vi "Positioncontrol_twomotor_pid_PMcheck.vi"() -> ()   [LabVIEW 2014]
uses:
  <vilib>/rvi/FXPMathLib/FxpSinAndCos/subVIs/nifxpmath_SinAndCos_SimConfig.ctl
  <vilib>/rvi/Emulation/niFpgaGetClockAttributes.vi
  <vilib>/rvi/Emulation/niFpgaSctlEmulationGetInTimedLoop.vi
  <vilib>/rvi/Emulation/niFpgaEmulationReportErrorSimple.vi
  <vilib>/rvi/Emulation/niFpgaProcessEmulError.vi
  <vilib>/rvi/FXPMathLib/FxpSinAndCos/simVIs/DllFxpSinAndCosTemp_sub.vi
  <vilib>/rvi/Emulation/niFpgaCriticalErrorInLSC.vi
  <vilib>/rvi/eio/common/nirviEmuTemplateMethod_errors.vi
  <vilib>/rvi/interface/RandomDataEmulation/nirviRandomDataMultiElementFPGAFIFO.vi
  <instcachedir>/0/nirviRandomDataMultiElementFPGAFIFO_AD0CFC12EF974623A9C2E4184BC062B2.lvgen/nirviRandomDataMultiElementFPGAFIFO_AD0CFC12EF974623A9C2E4184BC062B2_004.vi
  <vilib>/rvi/interface/RandomDataEmulation/niFpgaRandomDataHandleErrors.vi
  <vilib>/rvi/FXPMathLib/FxpSinAndCos/XNode/nifxpmath_SinAndCos.xnode
  <vilib>/eio/EIONode/EIONode.xnode
  <vilib>/rvi/FXPMathLib/FxpMul/XNode/nifxpmath_Multiplier.xnode
  <vilib>/rvi/FXPMathLib/FxpSub/XNode/nifxpmath_Sub.xnode
  <vilib>/rvi/FXPMathLib/FxpAdd/XNode/nifxpmath_Add.xnode
  <vilib>/rvi/Analysis/measure/butterworth/XNode/niFpgaButterworthFilter.xnode
  <vilib>/rvi/DataTransferAndStorage/Container/XNode/niFpgaContainer.xnode
  <vilib>/rvi/interface/RandomDataEmulation/nirviRandomDataFpgaMultiElementTemplate.vi
  <vilib>/rvi/FXPMathLib/sim/FxpSim.dll
panel:
  in  "AI loop wait (uSec)":u8=20
  in  "x_y 2 / x_y":bool
  in  "test stop/run":bool
  out "AI samp time (us) 3":u8
  in  "scaled coefficients_xy":i32[](array[numeric])=[-955995012, 2025731616, 1001305, -1023351008, 2092954700, 1034533]
  in  "scaled coefficients_xyd":i32[](array[numeric])=[-1013179863, 2085891919, 257442, -1048234864, 2120929620, 261767]
  in  "filter reset 2":bool
  out "AI diff samp time (us) 2":u8
  in  "AI diff loop wait (uSec) 2":u32
  out "Dy_d 2":fxp<+/-,25,15>
  out "Dp_d 2":fxp<+/-,25,15>
  in  "scaled coefficients_Dpd":i32[](array[numeric])=[780119100, 146811362]
  in  "scaled coefficients_Dyd":i32[](array[numeric])=[780119100, 146811362]
  in  "scaled coefficients_xpd":i32[](array[numeric])=[780119100, 146811362]
  out "xp_d 2":fxp<+/-,25,15>
  out "xy_d 2":fxp<+/-,25,15>
  out "AI samp time (us) 2":u8
  out "x_p 2":fxp<+/-,30,6> format="%.40g"
  in  "Linear Sensor Reset_y 2":bool
  out "x_y 2":fxp<+/-,30,6>
  in  "scaled coefficients_xp":i32[](array[numeric])=[1008310688, 32715568]
  in  "fyr_sin/cons":bool
  in  "fpr_sin/cons":bool
  in  "Sin_magnitude":fxp<+/-,12,8>
  in  "Sin_offset":fxp<+/-,12,8>
  out "fyr_sin":fxp<+/-,22,7> format="%.18g"
  out "fpr_sin":fxp<+/-,22,7> format="%.18g"
  in  "Sin_period(sec)":fxp<+,10,8> format="%.21g"
  in  "Time_reset":bool
  in  "coe_ini":bool
  out "fpt_i":fxp<+/-,25,11>
  out "fyt_i":fxp<+/-,25,11>
  out "time now":fxp<+/-,41,11>
  in  "D_comp/tune_p":bool
  in  "D_comp/tune_y":bool
  in  "kp t":fxp<+,15,8>
  in  "kp c":fxp<+,15,8>
  in  "Kpp gain":fxp<+,27,10>=0.40625
  in  "Kpp slope gain":fxp<+,20,1>=0.40625
  in  "Kdp 2":fxp<+,27,10>
  in  "Kip 2":fxp<+,27,10>
  in  "I_comp/tune_p":bool
  out "Kpp":fxp<+,12,6>
  out "Kdp":fxp<+,34,10> format="%.25g"
  out "Kip":fxp<+,27,10> format="%.21g"
  in  "tolerance_fp":fxp<+,12,2>=1.0
  in  "viscous_cons_p":fxp<+/-,20,10>
  in  "fcp":fxp<+/-,15,6>
  in  "fvp":fxp<+,20,12>
  in  "fv_coeff. p":fxp<+,13,1>
  in  "Dp_d_tol":fxp<+,20,12>
  in  "fstp":fxp<+/-,15,6>
  out "fpr":fxp<+/-,22,7> format="%.18g"
  out "Friction comp_p":fxp<+/-,20,10>
  out "Fp_PID":fxp<+/-,20,10>
  out "fp_tilde":fxp<+/-,26,11>
  out "xp_d":fxp<+/-,25,15>
  out "fpt_d":fxp<+/-,25,15>
  out "Dp_d":fxp<+/-,25,15>
  out "vd_p_F":fxp<+/-,20,5>
  out "vq_p_F":fxp<+/-,20,5> format="%.57g"
  in  "Stop motor_p":bool
  out "va_p":fxp<+/-,20,5> format="%.21g"
  out "vb_p":fxp<+/-,20,5> format="%.21g"
  out "omega_p":fxp<+/-,20,9>
  in  "Encoder Reset_p":bool
  out "Encoder Position_p":i32
  out "rad(NrTheta)_p":fxp<+/-,33,18> format="%.21g"
  out "Dp(mm)":fxp<+/-,22,7>
  in  "viscous_cons_y":fxp<+/-,20,10>
  in  "I_comp/tune_y":bool
  in  "fsty":fxp<+/-,15,6>
  out "Dy_d":fxp<+/-,25,15>
  out "fyr":fxp<+/-,22,7> format="%.18g"
  in  "Dy_d_tol":fxp<+,20,12>
  out "fy_tilde":fxp<+/-,26,11>
  out "fyt_d":fxp<+/-,25,15>
  in  "Kiy 2":fxp<+,27,10>
  in  "Kdy 2":fxp<+,27,10>
  in  "ky c":fxp<+,15,8>
  in  "ky t":fxp<+,15,8>
  out "Kiy":fxp<+,27,10> format="%.21g"
  in  "Kpy slope gain":fxp<+,20,1>=0.40625
  in  "Kpy gain":fxp<+,27,10>=0.40625
  in  "fv_coeff. y":fxp<+,13,1>
  out "Friction comp_y":fxp<+/-,20,10>
  in  "fcy":fxp<+/-,15,6>
  in  "fvy":fxp<+,20,12>
  out "xy_d":fxp<+/-,25,15>
  out "AI samp time (us)":u8
  out "x_p":fxp<+/-,30,6> format="%.40g"
  in  "Linear Sensor Reset_y":bool
  in  "kp":fxp<+,15,8>
  out "fp":fxp<+/-,20,10>
  in  "ky":fxp<+,15,8>
  out "fy":fxp<+/-,20,10>
  out "x_y":fxp<+/-,30,6> format="%.15g"
  out "Kdy":fxp<+,34,10> format="%.25g"
  out "Kpy":fxp<+,12,6>
  out "Fy_PID":fxp<+/-,20,10>
  in  "tolerance_fy":fxp<+,12,2>=1.0
  in  "Encoder Reset_y":bool
  out "Encoder Position_y":i32
  out "rad(NrTheta)_y":fxp<+/-,33,18> format="%.21g"
  out "Dy(mm)":fxp<+/-,22,7>
  out "omega_y":fxp<+/-,20,9>
  out "vq_y_F":fxp<+/-,20,5> format="%.57g"
  out "vd_y_F":fxp<+/-,20,5>
  in  "Stop motor_y":bool
  out "va_y":fxp<+/-,20,5> format="%.21g"
  out "vb_y":fxp<+/-,20,5> format="%.21g"
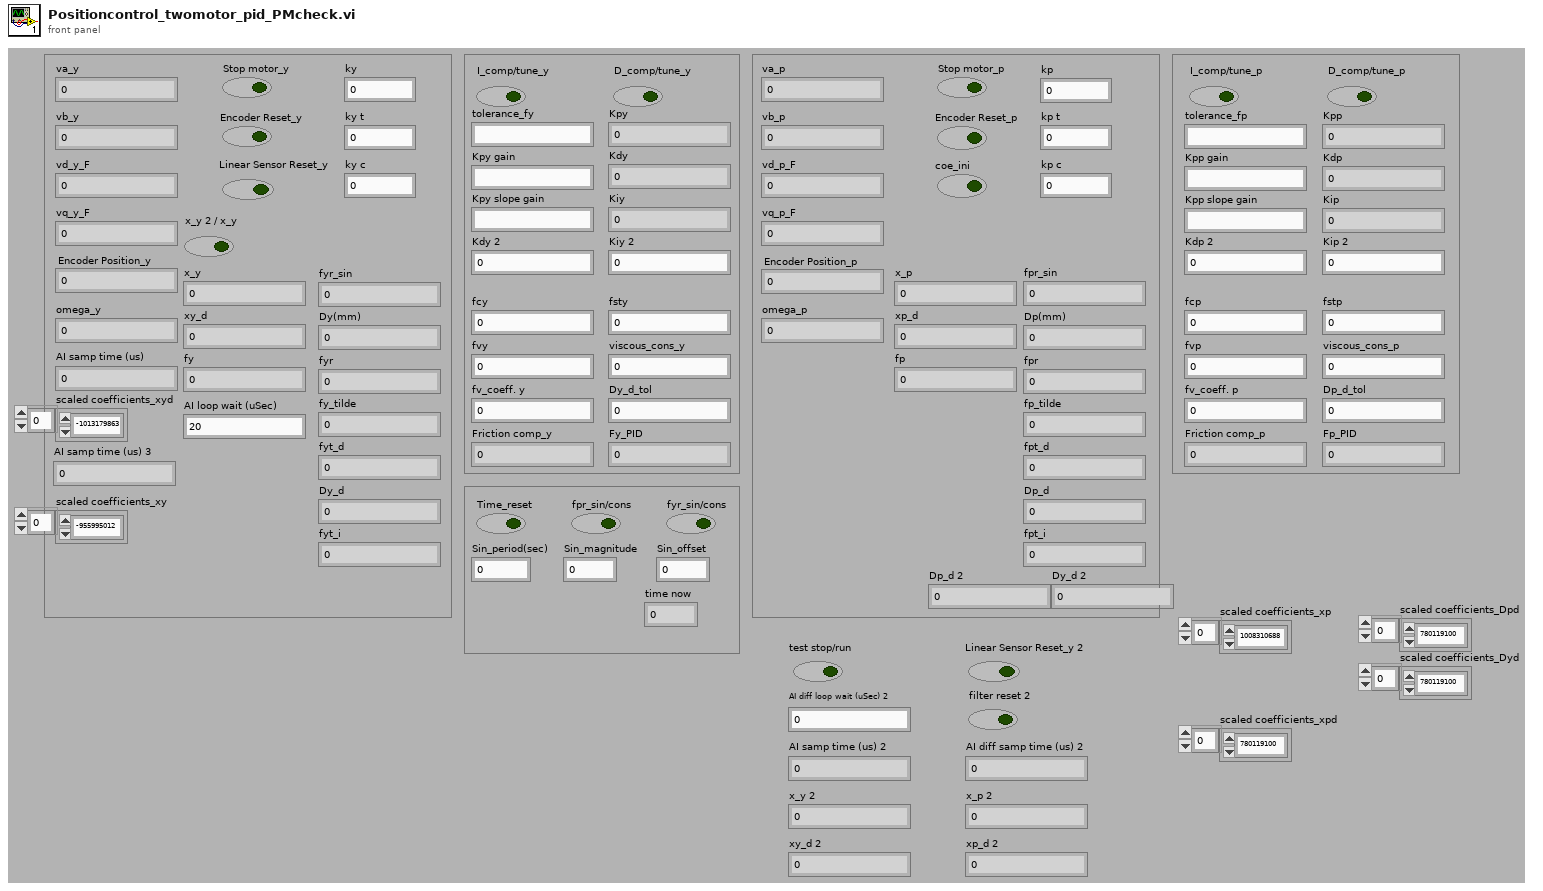
[diagram p1: front panel]
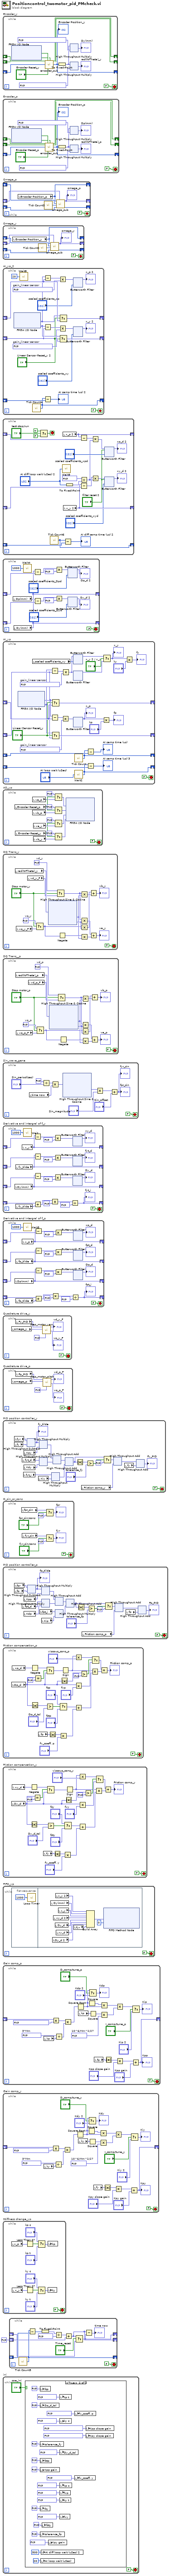
[diagram p0: block diagram]
diagram:
  n1 = while "Encoder_y" {
    shift-right: [w15] -> _
    shift-left: _ -> [w13]
    shift-right: [w14] -> _
    shift-left: _ -> [w12]
    shift-right: [w2] -> _
    shift-left: _ -> [w8]
    stop <- FALSE stop-if-true
    n2 = xnode "FPGA I/O Node"() -> ("Mod3/DIO2"=w11:bool, "Mod3/DIO3"=w10:bool)  [unwired: 2 in, 2 out]
    n3 = call "encoder_sub.vi"("A_pre"=w13, "B_pre"=w12, "Encoder Position_pre"=w8, "A input"=w11, "Encoder Position Reset"="Encoder Reset_y", "B input"=w10) -> ("A"=w15:bool, "B"=w14:bool, "Encoder Position (Counts)"=w2:i32)  [unwired: 19 in]
    "Encoder Position_y" <- w2
    n4 = To Fixed-Point(number=w2) -> (fixed-point=w5:fxp<+/-,18,18>)  [unwired: 1 in]
    n5 = xnode ("High Throughput Multiply")("x"=w5, "y"=fxp<+/-,15,-9> -0.0006049871444702148) -> ("x*y"=→"Dy(mm)":fxp<+/-,21,6>)
    n6 = xnode ("High Throughput Multiply")("x"=w5, "y"=fxp<+,24,0> 0.02499997615814209) -> ("x*y"=→"rad(NrTheta)_y":fxp<+/-,33,18>)
  }
  n7 = while "Encoder_p" {
    shift-right: [w30] -> _
    shift-left: _ -> [w28]
    shift-right: [w29] -> _
    shift-left: _ -> [w27]
    shift-right: [w17] -> _
    shift-left: _ -> [w23]
    stop <- FALSE stop-if-true
    n8 = xnode "FPGA I/O Node"() -> ("Mod3/DIO0"=w26:bool, "Mod3/DIO1"=w25:bool)  [unwired: 2 in, 2 out]
    n9 = call "encoder_sub.vi"("A_pre"=w28, "B_pre"=w27, "Encoder Position_pre"=w23, "A input"=w26, "Encoder Position Reset"="Encoder Reset_p", "B input"=w25) -> ("A"=w30:bool, "B"=w29:bool, "Encoder Position (Counts)"=w17:i32)  [unwired: 19 in]
    "Encoder Position_p" <- w17
    n10 = To Fixed-Point(number=w17) -> (fixed-point=w20:fxp<+/-,18,18>)  [unwired: 1 in]
    n11 = xnode ("High Throughput Multiply")("x"=w20, "y"=fxp<+/-,15,-9> -0.0006049871444702148) -> ("x*y"=→"Dp(mm)":fxp<+/-,21,6>)
    n12 = xnode ("High Throughput Multiply")("x"=w20, "y"=fxp<+,24,0> 0.02499997615814209) -> ("x*y"=→"rad(NrTheta)_p":fxp<+/-,33,18>)
  }
  n13 = while "Omega_p" {
    shift-right: [w39] -> _
    shift-left: _ -> [w38]
    shift-right: [w37] -> _
    shift-left: _ -> [w36]
    shift-right: [w34] -> _
    shift-left: _ -> [w35]
    stop <- FALSE stop-if-true
    n14 = local read "Encoder Position_p"() -> (w39:i32)
    n15 = call "Tick Count3"() -> ("Tick Count(Ticks)"=w32:u32)
    n16 = call "omega_sub.vi"("omega_pre"=w35, "ticks_m_pre"=w36, "ticks"=w32, "count_pre"=w38, "count"=w39) -> ("ticks_m"=w37:u32, "omega"=w34:fxp<+/-,20,9>)  [unwired: 5 in]
    "omega_p" <- w34
  }
  n17 = while "Omega_y" {
    shift-right: [w47] -> _
    shift-left: _ -> [w46]
    shift-right: [w45] -> _
    shift-left: _ -> [w44]
    shift-right: [w42] -> _
    shift-left: _ -> [w43]
    stop <- FALSE stop-if-true
    n18 = local read "Encoder Position_y"() -> (w47:i32)
    n19 = call "Tick Count2"() -> ("Tick Count(Ticks)"=w40:u32)
    n20 = call "omega_sub.vi"("omega_pre"=w43, "ticks_m_pre"=w44, "ticks"=w40, "count_pre"=w46, "count"=w47) -> ("ticks_m"=w45:u32, "omega"=w42:fxp<+/-,20,9>)  [unwired: 5 in]
    "omega_y" <- w42
  }
  n21 = while "AI_yp_2" {
    shift-right: [w68] -> _
    shift-left: _ -> [w69]
    shift-right: [w65] -> _
    shift-left: _ -> [w66]
    shift-right: [w63] -> _
    shift-left: _ -> [w62]
    stop <- FALSE stop-if-true
    w54 = fxp<+,25,5> 1.4694995880126953  # gain_linear sensor
    w59 = fxp<+,25,5> 1.5044002532958984  # gain_linear sensor
    n22 = xnode "FPGA I/O Node"() -> ("Mod1/AI0"=w64:fxp<+/-,20,5>, "Mod1/AI1"=w61:fxp<+/-,20,5>)  [unwired: 3 in, 3 out]
    n23 = call "Wait8"("Count(uSec)"=u8 20) -> ()  [unwired: 1 out]
    n24 = call "Tick Count4"() -> ("Tick Count(uSec)"=w68:u8)
    n25 = Subtract(x=w64, y=w66) -> (x-y=w58:fxp<+/-,21,6>)
    n26 = Subtract(x=w61, y=w62) -> (x-y=w60:fxp<+/-,21,6>)
    n27 = Subtract(x=w68, y=w69) -> (x-y=→"AI samp time (us) 2":u8)
    n28 = Multiply(x=w58, y=w54) -> (x*y=w56:fxp<+/-,30,6>)
    n29 = Multiply(x=w60, y=w59) -> (x*y=w55:fxp<+/-,30,6>)
    n30 = Select(t=w64, s="Linear Sensor Reset_y 2", f=w66) -> (s? t:f=w65:fxp<+/-,20,5>)
    n31 = Select(t=w61, s="Linear Sensor Reset_y 2", f=w62) -> (s? t:f=w63:fxp<+/-,20,5>)
    n32 = xnode "Butterworth Filter"("input data"=w56, "scaled coefficients"="scaled coefficients_xp") -> ("output data"=→"x_p 2":fxp<+/-,30,6>)  [unwired: 1 in]
    n33 = xnode "Butterworth Filter"("input data"=w55, "scaled coefficients"="scaled coefficients_xy") -> ("output data"=→"x_y 2":fxp<+/-,30,6>)  [unwired: 1 in]
  }
  n34 = while {
    shift-right: [w106] -> _
    shift-left: _ -> [w107]
    shift-right: [w104] -> _
    shift-left: _ -> [w105]
    shift-right: [w98] -> _
    shift-left: _ -> [w99]
    stop <- w86 stop-if-true
    n35 = Select(t=TRUE, s="test stop/run", f=FALSE) -> (s? t:f=w86:bool)
    n36 = call "Tick Count6"() -> ("Tick Count(uSec)"=w98:u8)
    n37 = call "Wait9"("Count(uSec)"="AI diff loop wait (uSec) 2") -> ()  [unwired: 1 out]
    n38 = local read "x_p 2"() -> (w106:fxp<+/-,30,6>)
    n39 = local read "x_y 2"() -> (w104:fxp<+/-,30,6>)
    n40 = Subtract(x=w98, y=w99) -> (x-y=→"AI diff samp time (us) 2":u8)
    n41 = To Fixed-Point(number="AI diff loop wait (uSec) 2") -> (fixed-point=w94:fxp<+,10,10>)  [unwired: 1 in]
    n42 = Subtract(x=w106, y=w107) -> (x-y=w109:fxp<+/-,31,7>)
    n43 = Subtract(x=w104, y=w105) -> (x-y=w108:fxp<+/-,31,7>)
    n44 = Divide(x=fxp<+,14,20> 1000000.0, y=w94) -> (x/y=w92:fxp<+,24,20>)
    n45 = Multiply(x=w109, y=w92) -> (x*y=w93:fxp<+/-,25,15>)
    n46 = Multiply(x=w108, y=w92) -> (x*y=w91:fxp<+/-,25,15>)
    n47 = xnode "Butterworth Filter"("input data"=w93, "reset"="filter reset 2", "scaled coefficients"="scaled coefficients_xpd") -> ("output data"=→"xp_d 2":fxp<+/-,25,15>)
    n48 = xnode "Butterworth Filter"("input data"=w91, "reset"="filter reset 2", "scaled coefficients"="scaled coefficients_xyd") -> ("output data"=→"xy_d 2":fxp<+/-,25,15>)
  }
  n49 = while {
    shift-right: [w132] -> _
    shift-left: _ -> [w133]
    shift-right: [w130] -> _
    shift-left: _ -> [w131]
    stop <- FALSE stop-if-true
    n50 = local read "Dp(mm)"() -> (w132:fxp<+/-,22,7>)
    n51 = local read "Dy(mm)"() -> (w130:fxp<+/-,22,7>)
    n52 = call "Wait4"("Count(uSec)"=u32 1000 ("Count(mSec)")) -> ()  [unwired: 1 out]
    n53 = Subtract(x=w132, y=w133) -> (x-y=w138:fxp<+/-,23,8>)
    n54 = Subtract(x=w130, y=w131) -> (x-y=w135:fxp<+/-,23,8>)
    n55 = Multiply(x=w138, y=fxp<+,10,10> 1000.0) -> (x*y=w139:fxp<+/-,25,15>)
    n56 = Multiply(x=w135, y=fxp<+,10,10> 1000.0) -> (x*y=w134:fxp<+/-,25,15>)
    n57 = xnode "Butterworth Filter"("input data"=w139, "scaled coefficients"="scaled coefficients_Dpd") -> ("output data"=→"Dp_d 2":fxp<+/-,25,15>)  [unwired: 1 in]
    n58 = xnode "Butterworth Filter"("input data"=w134, "scaled coefficients"="scaled coefficients_Dyd") -> ("output data"=→"Dy_d 2":fxp<+/-,25,15>)  [unwired: 1 in]
  }
  n59 = while "AI_yp" {
    shift-right: [w187] -> _
    shift-left: _ -> [w188]
    shift-right: [w183] -> _
    shift-left: _ -> [w184]
    shift-right: [w178] -> _
    shift-left: _ -> [w177]
    shift-right: [w166] -> _
    shift-left: _ -> [w165]
    stop <- FALSE stop-if-true
    w167 = fxp<+,25,5> 1.4694995880126953  # gain_linear sensor
    w174 = fxp<+,25,5> 1.5044002532958984  # gain_linear sensor
    n60 = xnode "FPGA I/O Node"() -> ("Mod1/AI0"=w180:fxp<+/-,20,5>, "Mod1/AI1"=w176:fxp<+/-,20,5>)  [unwired: 3 in, 3 out]
    n61 = local read "scaled coefficients_xy"() -> (w159:i32[])
    n62 = Subtract(x=w176, y=w177) -> (x-y=w175:fxp<+/-,21,6>)
    n63 = Subtract(x=w180, y=w184) -> (x-y=w171:fxp<+/-,21,6>)
    n64 = Select(t=w180, s="Linear Sensor Reset_y", f=w184) -> (s? t:f=w183:fxp<+/-,20,5>)
    n65 = Select(t=w176, s="Linear Sensor Reset_y", f=w177) -> (s? t:f=w178:fxp<+/-,20,5>)
    n66 = Multiply(x=w171, y=w167) -> (x*y=w169:fxp<+/-,30,6>)
    n67 = Multiply(x=w175, y=w174) -> (x*y=w158:fxp<+/-,30,6>)
    n68 = xnode "Butterworth Filter"("input data"=w158, "scaled coefficients"=w159) -> ("output data"=w161:fxp<+/-,30,6>)  [unwired: 1 in]
    n69 = xnode "Butterworth Filter"("input data"=w158) -> ("output data"=w160:fxp<+/-,30,6>)  [unwired: 2 in]
    n70 = xnode "Butterworth Filter"("input data"=w169) -> ("output data"=w168:fxp<+/-,30,6>)  [unwired: 2 in]
    "x_p" <- w168
    n71 = call "Wait2"("Count(uSec)"="AI loop wait (uSec)") -> ("Tick Count(uSec)"=w166:u8)
    n72 = call "Tick Count"() -> ("Tick Count(uSec)"=w187:u8)
    n73 = Subtract(x=w187, y=w188) -> (x-y=→"AI samp time (us)":u8)
    n74 = Subtract(x=w166, y=w165) -> (x-y=→"AI samp time (us) 3":u8)
    n75 = Multiply(x=w168, y="kp") -> (x*y=→"fp":fxp<+/-,20,10>)
    n76 = Select(t=w161, s="x_y 2 / x_y", f=w160) -> (s? t:f=w162:fxp<+/-,30,6>)
    "x_y" <- w162
    n77 = Multiply(x=w162, y="ky") -> (x*y=→"fy":fxp<+/-,20,10>)
  }
  n78 = while "AO_yp" {
    stop <- FALSE stop-if-true
    n79 = local read "Encoder Reset_p"() -> (w226:bool)
    n80 = local read "Encoder Reset_y"() -> (w215:bool)
    n81 = local read "va_p"() -> (w225:fxp<+/-,20,5>)
    n82 = local read "vb_p"() -> (w224:fxp<+/-,20,5>)
    n83 = local read "va_y"() -> (w216:fxp<+/-,20,5>)
    n84 = local read "vb_y"() -> (w217:fxp<+/-,20,5>)
    n85 = Select(t=fxp<+/-,20,5> 5.0 ("Mod2/AO4"), s=w226, f=w225) -> (s? t:f=w221:fxp<+/-,20,5>)
    n86 = Select(t=fxp<+/-,20,5> 0.0 ("Mod2/AO4"), s=w226, f=w224) -> (s? t:f=w220:fxp<+/-,20,5>)
    n87 = Select(t=fxp<+/-,20,5> 5.0 ("Mod2/AO4"), s=w215, f=w216) -> (s? t:f=w214:fxp<+/-,20,5>)
    n88 = Select(t=fxp<+/-,20,5> 0.0 ("Mod2/AO4"), s=w215, f=w217) -> (s? t:f=w213:fxp<+/-,20,5>)
    n89 = xnode "FPGA I/O Node"("Mod2/AO0"=w221, "Mod2/AO1"=w220, "Mod2/AO2"=w214, "Mod2/AO3"=w213) -> ()  [unwired: 4 in, 4 out]
  }
  n90 = while "DQ Trans_y" {
    stop <- FALSE stop-if-true
    w233 = fxp<+/-,20,5> 0.0  # vq_y
    w231 = fxp<+/-,20,5> 0.0  # vd_y
    n91 = local read "rad(NrTheta)_y"() -> (w244:fxp<+/-,33,18>)
    n92 = local read "vq_y_F"() -> (w229:fxp<+/-,20,5>)
    n93 = local read "vd_y_F"() -> (w230:fxp<+/-,20,5>)
    n94 = Select(t=w233, s="Stop motor_y", f=w229) -> (s? t:f=w234:fxp<+/-,20,5>)
    n95 = xnode "High Throughput Sine & Cosine"("x (pi)"=w244) -> ("sin(x)"=w235:fxp<+/-,17,2>, "cos(x)"=w236:fxp<+/-,17,2>)
    n96 = Select(t=w231, s="Stop motor_y", f=w230) -> (s? t:f=w232:fxp<+/-,20,5>)
    n97 = Negate(x=w234) -> (-x=w243:fxp<+/-,21,6>)
    n98 = Multiply(x=w232, y=w235) -> (x*y=w239:fxp<+/-,20,5>)
    n99 = Multiply(x=w232, y=w236) -> (x*y=w242:fxp<+/-,20,5>)
    n100 = Multiply(x=w234, y=w236) -> (x*y=w238:fxp<+/-,20,5>)
    n101 = Multiply(x=w243, y=w235) -> (x*y=w241:fxp<+/-,20,5>)
    n102 = Add(x=w238, y=w239) -> (x+y=→"vb_y":fxp<+/-,20,5>)
    n103 = Add(x=w242, y=w241) -> (x+y=→"va_y":fxp<+/-,20,5>)
  }
  n104 = while "DQ Trans__p" {
    stop <- FALSE stop-if-true
    w283 = fxp<+/-,20,5> 0.0  # vq_p
    w281 = fxp<+/-,20,5> 0.0  # vd_p
    n105 = local read "rad(NrTheta)_p"() -> (w292:fxp<+/-,33,18>)
    n106 = local read "vq_p_F"() -> (w279:fxp<+/-,20,5>)
    n107 = local read "vd_p_F"() -> (w280:fxp<+/-,20,5>)
    n108 = Select(t=w283, s="Stop motor_p", f=w279) -> (s? t:f=w284:fxp<+/-,20,5>)
    n109 = xnode "High Throughput Sine & Cosine"("x (pi)"=w292) -> ("sin(x)"=w285:fxp<+/-,17,2>, "cos(x)"=w286:fxp<+/-,17,2>)
    n110 = Select(t=w281, s="Stop motor_p", f=w280) -> (s? t:f=w282:fxp<+/-,20,5>)
    n111 = Negate(x=w284) -> (-x=w291:fxp<+/-,21,6>)
    n112 = Multiply(x=w282, y=w285) -> (x*y=w288:fxp<+/-,20,5>)
    n113 = Multiply(x=w282, y=w286) -> (x*y=w290:fxp<+/-,20,5>)
    n114 = Multiply(x=w284, y=w286) -> (x*y=w287:fxp<+/-,20,5>)
    n115 = Multiply(x=w291, y=w285) -> (x*y=w289:fxp<+/-,20,5>)
    n116 = Add(x=w287, y=w288) -> (x+y=→"vb_p":fxp<+/-,20,5>)
    n117 = Add(x=w290, y=w289) -> (x+y=→"va_p":fxp<+/-,20,5>)
  }
  n118 = while "Sin_wave_gene" {
    stop <- FALSE stop-if-true
    n119 = local read "time now"() -> (w333:fxp<+/-,41,11>)
    n120 = Divide(x=fxp<+,10,8> 2.0, y="Sin_period(sec)") -> (x/y=w332:fxp<+/-,20,11>)
    n121 = Multiply(x=w332, y=w333) -> (x*y=w331:fxp<+/-,25,11>)
    n122 = xnode "High Throughput Sine & Cosine"("x (pi)"=w331) -> ("sin(x)"=w329:fxp<+/-,17,2>)  [unwired: 1 out]
    n123 = Multiply(x=w329, y="Sin_magnitude") -> (x*y=w327:fxp<+/-,20,8>)
    n124 = Add(x=w327, y="Sin_offset") -> (x+y=→"fyr_sin" →"fpr_sin":fxp<+/-,22,7>)
  }
  n125 = while "Derivative and intergral of f_y" {
    shift-right: [w386] -> _
    shift-left: _ -> [w385]
    shift-right: [w382] -> _
    shift-left: _ -> [w383]
    shift-right: [w375] -> _
    shift-left: _ -> [w374]
    shift-right: [w367] -> _
    shift-left: _ -> [w368]
    stop <- FALSE stop-if-true
    n126 = local read "Dy(mm)"() -> (w375:fxp<+/-,22,7>)
    n127 = local read "fy_tilde"() -> (w382:fxp<+/-,26,11>)
    n128 = local read "fy_tilde"() -> (w369:fxp<+/-,26,11>)
    n129 = local read "x_y"() -> (w386:fxp<+/-,30,6>)
    n130 = call "Wait"("Count(uSec)"=u32 1000 ("Count(mSec)")) -> ()  [unwired: 1 out]
    n131 = Subtract(x=w386, y=w385) -> (x-y=w388:fxp<+/-,31,7>)
    n132 = Subtract(x=w382, y=w383) -> (x-y=w379:fxp<+/-,27,12>)
    n133 = Subtract(x=w375, y=w374) -> (x-y=w377:fxp<+/-,23,8>)
    n134 = Add(x=w368, y=w369) -> (x+y=w370:fxp<+/-,27,12>)
    n135 = Multiply(x=w370, y=fxp<+/-,22,12> 0.5) -> (x*y=w372:fxp<+/-,25,15>)
    n136 = Multiply(x=w388, y=fxp<+,10,10> 1000.0) -> (x*y=w387:fxp<+/-,25,15>)
    n137 = Multiply(x=w379, y=fxp<+,10,10> 1000.0) -> (x*y=w381:fxp<+/-,25,15>)
    n138 = Multiply(x=w377, y=fxp<+,10,10> 1000.0) -> (x*y=w366:fxp<+/-,25,15>)
    n139 = Divide(x=w372, y=fxp<+/-,25,15> 1000.0) -> (x/y=w367:fxp<+/-,25,11>)
    "fyt_i" <- w367
    n140 = xnode "Butterworth Filter"("input data"=w387) -> ("output data"=→"xy_d":fxp<+/-,25,15>)  [unwired: 2 in]
    n141 = xnode "Butterworth Filter"("input data"=w381) -> ("output data"=→"fyt_d":fxp<+/-,25,15>)  [unwired: 2 in]
    n142 = xnode "Butterworth Filter"("input data"=w366) -> ("output data"=→"Dy_d":fxp<+/-,25,15>)  [unwired: 2 in]
  }
  n143 = while "Derivative and intergral of f_p" {
    shift-right: [w434] -> _
    shift-left: _ -> [w433]
    shift-right: [w430] -> _
    shift-left: _ -> [w431]
    shift-right: [w423] -> _
    shift-left: _ -> [w422]
    shift-right: [w415] -> _
    shift-left: _ -> [w416]
    stop <- FALSE stop-if-true
    n144 = local read "Dp(mm)"() -> (w423:fxp<+/-,22,7>)
    n145 = local read "fp_tilde"() -> (w430:fxp<+/-,26,11>)
    n146 = local read "fp_tilde"() -> (w421:fxp<+/-,26,11>)
    n147 = local read "x_p"() -> (w434:fxp<+/-,30,6>)
    n148 = call "Wait3"("Count(uSec)"=u32 1000 ("Count(mSec)")) -> ()  [unwired: 1 out]
    n149 = Subtract(x=w434, y=w433) -> (x-y=w436:fxp<+/-,31,7>)
    n150 = Subtract(x=w430, y=w431) -> (x-y=w427:fxp<+/-,27,12>)
    n151 = Subtract(x=w423, y=w422) -> (x-y=w425:fxp<+/-,23,8>)
    n152 = Add(x=w416, y=w421) -> (x+y=w420:fxp<+/-,27,12>)
    n153 = Multiply(x=w420, y=fxp<+/-,22,12> 0.5) -> (x*y=w418:fxp<+/-,25,15>)
    n154 = Multiply(x=w436, y=fxp<+,10,10> 1000.0) -> (x*y=w435:fxp<+/-,25,15>)
    n155 = Multiply(x=w427, y=fxp<+,10,10> 1000.0) -> (x*y=w429:fxp<+/-,25,15>)
    n156 = Multiply(x=w425, y=fxp<+,10,10> 1000.0) -> (x*y=w414:fxp<+/-,25,15>)
    n157 = Divide(x=w418, y=fxp<+/-,25,15> 1000.0) -> (x/y=w415:fxp<+/-,25,11>)
    "fpt_i" <- w415
    n158 = xnode "Butterworth Filter"("input data"=w435) -> ("output data"=→"xp_d":fxp<+/-,25,15>)  [unwired: 2 in]
    n159 = xnode "Butterworth Filter"("input data"=w429) -> ("output data"=→"fpt_d":fxp<+/-,25,15>)  [unwired: 2 in]
    n160 = xnode "Butterworth Filter"("input data"=w414) -> ("output data"=→"Dp_d":fxp<+/-,25,15>)  [unwired: 2 in]
  }
  n161 = while "Quadrature drive_y" {
    stop <- FALSE stop-if-true
    n162 = local read "omega_y"() -> (w464:fxp<+/-,20,9>)
    n163 = local read "Fy_PID"() -> (w465:fxp<+/-,20,10>)
    n164 = call "step_motor_yaw.vi"("F_Threshold"=fxp<+,12,12> 10.0, "omega_y"=w464, "F"=w465) -> ("vq_F"=→"vq_y_F":fxp<+/-,20,5>, "vd_F"=→"vd_y_F":fxp<+/-,20,5>)  [unwired: 7 in]
  }
  n165 = while "Quadrature drive_p" {
    stop <- FALSE stop-if-true
    n166 = local read "omega_p"() -> (w469:fxp<+/-,20,9>)
    n167 = local read "Fp_PID"() -> (w471:fxp<+/-,20,10>)
    n168 = call "step_motor_pitch.vi"("F_Threshold"=fxp<+,12,12> 10.0, "omega_p"=w469, "F"=w471) -> ("vq_F"=→"vq_p_F":fxp<+/-,20,5>, "vd_F"=→"vd_p_F":fxp<+/-,20,5>)  [unwired: 7 in]
  }
  n169 = while "PID position controller_y" {
    stop <- FALSE stop-if-true
    n170 = local read "fyr"() -> (w486:fxp<+/-,22,7>)
    n171 = local read "fy"() -> (w473:fxp<+/-,20,10>)
    n172 = local read "fyt_d"() -> (w482:fxp<+/-,25,15>)
    n173 = local read "fyt_i"() -> (w480:fxp<+/-,25,11>)
    n174 = local read "Kpy"() -> (w484:fxp<+,12,6>)
    n175 = local read "Kdy"() -> (w483:fxp<+,34,10>)
    n176 = xnode "High Throughput Subtract"("x"=w486, "y"=w473) -> ("x-y"=w485:fxp<+/-,26,11>)
    "fy_tilde" <- w485
    n177 = local read "Kiy"() -> (w481:fxp<+,27,10>)
    n178 = xnode ("High Throughput Multiply")("x"=w485, "y"=w484) -> ("x*y"=w479:fxp<+/-,38,17>)
    n179 = xnode ("High Throughput Multiply")("x"=w482, "y"=w483) -> ("x*y"=w478:fxp<+/-,59,25>)
    n180 = xnode ("High Throughput Multiply")("x"=w480, "y"=w481) -> ("x*y"=w477:fxp<+/-,52,21>)
    n181 = xnode ("High Throughput Add")("x"=w479, "y"=w478) -> ("x+y"=w476:fxp<+/-,60,26>)
    n182 = xnode ("High Throughput Add")("x"=w476, "y"=w477) -> ("x+y"=w475:fxp<+/-,20,10>)
    n183 = Absolute Value(x=w475) -> (abs(x)=w493:fxp<+,20,10>)
    n184 = local read "Friction comp_y"() -> (w487:fxp<+/-,20,10>)
    n185 = Greater?(x=w493, y="tolerance_fy") -> (0:w492:bool)
    n186 = Select(t=w475, s=w492, f=fxp<+/-,20,10> 0.0) -> (s? t:f=w489:fxp<+/-,20,10>)
    n187 = xnode ("High Throughput Add")("x"=w489, "y"=w487) -> ("x+y"=w488:fxp<+/-,20,10>)
    n188 = local read "fy"() -> (w490:fxp<+/-,20,10>)
    n189 = xnode ("High Throughput Add")("x"=w488, "y"=w490) -> ("x+y"=→"Fy_PID":fxp<+/-,20,10>)
  }
  n190 = while "D_sin_or_cons" {
    stop <- FALSE stop-if-true
    n191 = local read "fpr_sin"() -> (w500:fxp<+/-,22,7>)
    n192 = local read "fyr_sin"() -> (w499:fxp<+/-,22,7>)
    n193 = Select(t=w500, s="fpr_sin/cons", f=fxp<+/-,22,7> 0.0) -> (s? t:f=→"fpr":fxp<+/-,22,7>)
    n194 = Select(t=w499, s="fyr_sin/cons", f=fxp<+/-,22,7> 0.0) -> (s? t:f=→"fyr":fxp<+/-,22,7>)
  }
  n195 = while "PID position controller_p" {
    stop <- FALSE stop-if-true
    n196 = local read "fpr"() -> (w516:fxp<+/-,22,7>)
    n197 = local read "fp"() -> (w505:fxp<+/-,20,10>)
    n198 = local read "fpt_d"() -> (w519:fxp<+/-,25,15>)
    n199 = local read "Kpp"() -> (w517:fxp<+,12,6>)
    n200 = local read "Kdp"() -> (w518:fxp<+,34,10>)
    n201 = xnode "High Throughput Subtract"("x"=w516, "y"=w505) -> ("x-y"=w512:fxp<+/-,26,11>)
    "fp_tilde" <- w512
    n202 = local read "fpt_i"() -> (w521:fxp<+/-,25,11>)
    n203 = xnode ("High Throughput Multiply")("x"=w512, "y"=w517) -> ("x*y"=w522:fxp<+/-,38,17>)
    n204 = xnode ("High Throughput Multiply")("x"=w519, "y"=w518) -> ("x*y"=w523:fxp<+/-,59,25>)
    n205 = local read "Kip"() -> (w520:fxp<+,27,10>)
    n206 = xnode ("High Throughput Add")("x"=w522, "y"=w523) -> ("x+y"=w525:fxp<+/-,60,26>)
    n207 = xnode ("High Throughput Multiply")("x"=w521, "y"=w520) -> ("x*y"=w524:fxp<+/-,52,21>)
    n208 = xnode ("High Throughput Add")("x"=w525, "y"=w524) -> ("x+y"=w526:fxp<+/-,20,10>)
    n209 = Absolute Value(x=w526) -> (abs(x)=w513:fxp<+,20,10>)
    n210 = local read "Friction comp_p"() -> (w509:fxp<+/-,20,10>)
    n211 = Greater?(x=w513, y="tolerance_fp") -> (0:w514:bool)
    n212 = Select(t=w526, s=w514, f=fxp<+/-,20,10> 0.0) -> (s? t:f=w510:fxp<+/-,20,10>)
    n213 = xnode ("High Throughput Add")("x"=w510, "y"=w509) -> ("x+y"=w507:fxp<+/-,20,10>)
    n214 = local read "fp"() -> (w508:fxp<+/-,20,10>)
    n215 = xnode ("High Throughput Add")("x"=w507, "y"=w508) -> ("x+y"=→"Fp_PID":fxp<+/-,20,10>)
  }
  n216 = while "Friction compensation_p" {
    stop <- FALSE stop-if-true
    n217 = local read "Dp_d"() -> (w534:fxp<+/-,25,15>)
    n218 = local read "xp_d"() -> (w529:fxp<+/-,25,15>)
    n219 = Negate(x=w529) -> (-x=w528:fxp<+/-,26,16>)
    n220 = Absolute Value(x=w534) -> (abs(x)=w547:fxp<+,25,15>)
    n221 = Equal?(x=w534, y=fxp<+/-,25,15> 0.0) -> (x = y?=w535:bool)
    n222 = local read "fp"() -> (w552:fxp<+/-,20,10>)
    n223 = Greater?(x=w547, y="Dp_d_tol") -> (0:w546:bool)
    n224 = Select(t=w528, s=w535, f=w534) -> (s? t:f=w533:fxp<+/-,26,16>)
    n225 = Absolute Value(x=w552) -> (abs(x)=w553:fxp<+,20,10>)
    n226 = Select(t="fcp", s=w546, f="fstp") -> (s? t:f=w544:fxp<+/-,15,6>)
    n227 = Multiply(x=w553, y="fv_coeff. p") -> (x*y=w551:fxp<+/-,20,10>)
    n228 = Absolute Value(x=w534) -> (abs(x)=w541:fxp<+,25,15>)
    n229 = Sign(1:w533) -> (0:w532:fxp<+/-,2,2>)
    n230 = Multiply(x=w532, y="viscous_cons_p") -> (x*y=w537:fxp<+/-,20,10>)
    n231 = Multiply(x=w534, y="fvp") -> (x*y=w539:fxp<+/-,20,10>)
    n232 = Add(x=w544, y=w551) -> (x+y=w550:fxp<+/-,20,10>)
    n233 = Greater?(x=w541, y=fxp<+/-,25,15> 25.0) -> (0:w540:bool)
    n234 = Multiply(x=w532, y=w550) -> (x*y=w549:fxp<+/-,20,10>)
    n235 = Select(t=w537, s=w540, f=w539) -> (s? t:f=w538:fxp<+/-,20,10>)
    n236 = Add(x=w538, y=w549) -> (x+y=→"Friction comp_p":fxp<+/-,20,10>)
  }
  n237 = while "Friction compensation_y" {
    stop <- FALSE stop-if-true
    n238 = local read "Dy_d"() -> (w561:fxp<+/-,25,15>)
    n239 = local read "xy_d"() -> (w558:fxp<+/-,25,15>)
    n240 = Negate(x=w558) -> (-x=w557:fxp<+/-,26,16>)
    n241 = Absolute Value(x=w561) -> (abs(x)=w575:fxp<+,25,15>)
    n242 = Equal?(x=w561, y=fxp<+/-,25,15> 0.0) -> (x = y?=w562:bool)
    n243 = local read "fy"() -> (w581:fxp<+/-,20,10>)
    n244 = Select(t=w557, s=w562, f=w561) -> (s? t:f=w560:fxp<+/-,26,16>)
    n245 = Greater?(x=w575, y="Dy_d_tol") -> (0:w574:bool)
    n246 = Absolute Value(x=w581) -> (abs(x)=w582:fxp<+,20,10>)
    n247 = Multiply(x=w582, y="fv_coeff. y") -> (x*y=w579:fxp<+/-,20,10>)
    n248 = Select(t="fcy", s=w574, f="fsty") -> (s? t:f=w572:fxp<+/-,15,6>)
    n249 = Absolute Value(x=w561) -> (abs(x)=w569:fxp<+,25,15>)
    n250 = Sign(1:w560) -> (0:w559:fxp<+/-,2,2>)
    n251 = Multiply(x=w559, y="viscous_cons_y") -> (x*y=w564:fxp<+/-,20,10>)
    n252 = Multiply(x=w561, y="fvy") -> (x*y=w567:fxp<+/-,20,10>)
    n253 = Add(x=w572, y=w579) -> (x+y=w578:fxp<+/-,20,10>)
    n254 = Greater?(x=w569, y=fxp<+/-,25,15> 25.0) -> (0:w568:bool)
    n255 = Multiply(x=w559, y=w578) -> (x*y=w577:fxp<+/-,20,10>)
    n256 = Select(t=w564, s=w568, f=w567) -> (s? t:f=w566:fxp<+/-,20,10>)
    n257 = Add(x=w566, y=w577) -> (x+y=→"Friction comp_y":fxp<+/-,20,10>)
  }
  n258 = while "FIFO_yp" {
    stop <- FALSE stop-if-true
    n259 = flat-sequence {
      frame #0 {
        n260 = call "Loop Timer"("Count(uSec)"=u32 1000 ("Loop Period (usec)")) -> ()  [unwired: 1 out]
      }
      frame #1 {
        n261 = local read "Dy(mm)"() -> (w594:fxp<+/-,22,7>)
        n262 = local read "Dy_d 2"() -> (w589:fxp<+/-,25,15>)
        n263 = local read "xy_d 2"() -> (w592:fxp<+/-,25,15>)
        n264 = local read "Dy_d"() -> (w591:fxp<+/-,25,15>)
        n265 = local read "x_y 2"() -> (w597:fxp<+/-,30,6>)
        n266 = local read "xy_d"() -> (w590:fxp<+/-,25,15>)
        n267 = local read "x_y"() -> (w593:fxp<+/-,30,6>)
        n268 = local read "fyr"() -> (w588:fxp<+/-,22,7>)
        n269 = Build Array(w597, w594, w593, w592, w591, w590, w589, w588) -> (w596:fxp<+/-,39,15>[])
        n270 = xnode ("FIFO Method Node")("Element"=w596, "Timeout"=0) -> ()  [unwired: 1 in, 2 out]
      }
    }
  }
  n271 = while "Gain comp_p" {
    shift-right: [w602] -> _
    shift-left: _ -> [w621]
    stop <- FALSE stop-if-true
    w609 = fxp<+,14,7> 111.8125  # 10^6/Mm^2/27
    w624 = fxp<+,14,7> 54.6015625  # 3*Mm
    n272 = local read "kp"() -> (w623:fxp<+,15,8>)
    n273 = Multiply(x=w621, y=fxp<+,12,-6> 0.00099945068359375) -> (x*y=w620:fxp<+,24,0>)
    n274 = Divide(x=w624, y=w623) -> (x/y=w619:fxp<+,23,7>)
    n275 = Multiply(x=w620, y=w619) -> (x*y=w618:fxp<+,32,0>)
    n276 = Square Root(x=w618) -> (sqrt(x)=w605:fxp<+,26,2>)
    n277 = local read "kp"() -> (w610:fxp<+,15,8>)
    n278 = Square(x=w605) -> (x^2=w612:fxp<+,27,3>)
    n279 = Select(t=w605, s="D_comp/tune_p", f="Kdp 2") -> (s? t:f=→"Kdp":fxp<+,34,10>)
    n280 = Square(x=w610) -> (x^2=w608:fxp<+,30,16>)
    n281 = local read "fp"() -> (w615:fxp<+/-,20,10>)
    n282 = Multiply(x=w612, y=w605) -> (x*y=w611:fxp<+,27,3>)
    n283 = Multiply(x=w608, y=w609) -> (x*y=w607:fxp<+,44,20>)
    n284 = Absolute Value(x=w615) -> (abs(x)=w616:fxp<+,20,10>)
    n285 = Multiply(x=w611, y=w607) -> (x*y=w604:fxp<+,27,10>)
    n286 = Multiply(x=w616, y="Kpp slope gain") -> (x*y=w614:fxp<+,12,4>)
    n287 = Add(x=w614, y="Kpp gain") -> (x+y=w602:fxp<+,12,6>)
    "Kpp" <- w602
    n288 = Select(t=w604, s="I_comp/tune_p", f="Kip 2") -> (s? t:f=→"Kip":fxp<+,27,10>)
  }
  n289 = while "Gain comp_y" {
    shift-right: [w640] -> _
    shift-left: _ -> [w649]
    stop <- FALSE stop-if-true
    w636 = fxp<+,14,7> 111.8125  # 10^6/Mm^2/27
    w652 = fxp<+,14,7> 54.6015625  # 3*Mm
    n290 = local read "ky"() -> (w651:fxp<+,15,8>)
    n291 = Multiply(x=w649, y=fxp<+,12,-6> 0.00099945068359375) -> (x*y=w648:fxp<+,24,0>)
    n292 = Divide(x=w652, y=w651) -> (x/y=w647:fxp<+,23,7>)
    n293 = Multiply(x=w648, y=w647) -> (x*y=w646:fxp<+,32,0>)
    n294 = Square Root(x=w646) -> (sqrt(x)=w631:fxp<+,26,2>)
    n295 = local read "ky"() -> (w637:fxp<+,15,8>)
    n296 = Square(x=w631) -> (x^2=w639:fxp<+,27,3>)
    n297 = Select(t=w631, s="D_comp/tune_y", f="Kdy 2") -> (s? t:f=→"Kdy":fxp<+,34,10>)
    n298 = Square(x=w637) -> (x^2=w635:fxp<+,30,16>)
    n299 = local read "fy"() -> (w643:fxp<+/-,20,10>)
    n300 = Multiply(x=w639, y=w631) -> (x*y=w638:fxp<+,27,3>)
    n301 = Multiply(x=w635, y=w636) -> (x*y=w634:fxp<+,44,20>)
    n302 = Absolute Value(x=w643) -> (abs(x)=w644:fxp<+,20,10>)
    n303 = Multiply(x=w638, y=w634) -> (x*y=w629:fxp<+,27,10>)
    n304 = Multiply(x=w644, y="Kpy slope gain") -> (x*y=w642:fxp<+,12,4>)
    n305 = Add(x=w642, y="Kpy gain") -> (x+y=w640:fxp<+,12,6>)
    "Kpy" <- w640
    n306 = Select(t=w629, s="I_comp/tune_y", f="Kiy 2") -> (s? t:f=→"Kiy":fxp<+,27,10>)
  }
  n307 = while "Stiffness change_yp" {
    stop <- FALSE stop-if-true
    n308 = local read "x_p"() -> (w654:fxp<+/-,30,6>)
    n309 = local read "x_y"() -> (w664:fxp<+/-,30,6>)
    n310 = Less Than 0?(x=w654) -> (x < 0?=w655:bool)
    n311 = Less Than 0?(x=w664) -> (x < 0?=w663:bool)
    n312 = Select(t="kp c", s=w655, f="kp t") -> (s? t:f=w656:fxp<+,15,8>)
    n313 = Select(t="ky c", s=w663, f="ky t") -> (s? t:f=w662:fxp<+,15,8>)
    n314 = local write "kp"(w656) -> ()
    n315 = local write "ky"(w662) -> ()
  }
  n316 = while "ini" {
    stop <- FALSE stop-if-true
    n317 = case shown="True" "coe_ini" {
      frame False {
      }
      frame True {
        n318 = local write "fcp"(fxp<+/-,15,6> 6.0 ("fcp")) -> ()
        n319 = local write "Dp_d_tol"(fxp<+,20,12> 3.0 ("Dp_d_tol")) -> ()
        n320 = local write "tolerance_fy"(fxp<+,12,2> 1.0 ("tolerance_y")) -> ()
        n321 = local write "fstp"(fxp<+/-,15,6> 8.0 ("fstp")) -> ()
        n322 = local write "Kpp gain"(fxp<+,27,10> 3.0 ("Kpp gain")) -> ()
        n323 = local write "fcy"(fxp<+/-,15,6> 6.0 ("fcy")) -> ()
        n324 = local write "tolerance_fp"(fxp<+,12,2> 1.0 ("tolerance_p")) -> ()
        n325 = local write "AI loop wait (uSec)"(u8 20 ("AI loop wait (uSec)")) -> ()
        n326 = local write "AI diff loop wait (uSec) 2"(u32 500 ("AI diff loop wait (uSec) 2")) -> ()
        n327 = local write "fsty"(fxp<+/-,15,6> 12.0 ("fsty")) -> ()
        n328 = local write "Kpy gain"(fxp<+,27,10> 2.296875 ("Kpy gain")) -> ()
        n329 = local write "kp t"(fxp<+,15,8> 31.8046875 ("kp t")) -> ()
        n330 = local write "ky c"(fxp<+,15,8> 34.0234375 ("kp c")) -> ()
        n331 = local write "Dy_d_tol"(fxp<+,20,12> 0.1015625 ("Dy_d_tol")) -> ()
        n332 = local write "kp c"(fxp<+,15,8> 36.2421875 ("kp c")) -> ()
        n333 = local write "fvp"(fxp<+,20,12> 0.19921875 ("fvp")) -> ()
        n334 = local write "ky t"(fxp<+,15,8> 33.3359375 ("ky")) -> ()
        n335 = local write "fvy"(fxp<+,20,12> 0.19921875 ("fvy")) -> ()
        n336 = local write "fv_coeff. p"(fxp<+,13,1> 0.14990234375 ("fv_coeff. p")) -> ()
        n337 = local write "fv_coeff. y"(fxp<+,13,1> 0.14990234375 ("fv_coeff. y")) -> ()
        n338 = local write "Kpp slope gain"(fxp<+,20,1> 0.14999961853027344 ("Kpp slope gain")) -> ()
        n339 = local write "Kpy slope gain"(fxp<+,20,1> 0.14999961853027344 ("Kpy slope gain")) -> ()
      }
    }
  }
  n340 = while {
    shift-right: [w700] -> _
    shift-left: _ -> [w701]
    shift-right: [w693] -> _
    shift-left: fxp<+,36,6> 0.0 -> [w699]
    shift-right: [w691] -> _
    shift-left: _ -> [w692]
    stop <- FALSE stop-if-true
    n341 = call "Tick Count5"() -> ("Tick Count(uSec)"=w700:u8)
    n342 = Subtract(x=w700, y=w701) -> (x-y=w697:u8)
    n343 = To Fixed-Point(number=w697) -> (fixed-point=w696:fxp<+,8,8>)  [unwired: 1 in]
    n344 = Divide(x=w696, y=fxp<+,14,20> 1000000.0) -> (x/y=w695:fxp<+,15,-15>)
    n345 = Add(x=w695, y=w699) -> (x+y=w693:fxp<+,40,10>)
    n346 = Select(t=w693, s="Time_reset", f=w692) -> (s? t:f=w691:fxp<+,40,10>)
    n347 = Subtract(x=w693, y=w691) -> (x-y=→"time now":fxp<+/-,41,11>)
  }
